vi "GUIQueueCluster.vi"() -> ()   [LabVIEW 2017]
uses:
  GUIQueueCluster.ctl
  GUIMessage.ctl
panel:
  in  "GUIQueueCluster":T1
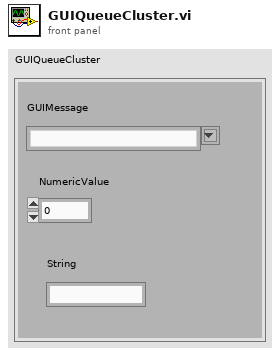
[diagram p1: front panel]
types:
  T1 = typedef "GUIQueueCluster.ctl" = cluster{"GUIMessage":T2, "NumericValue":dbl, "String":string}
  T2 = typedef "GUIMessage.ctl" = string
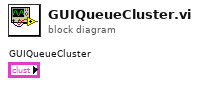
[diagram p0: block diagram]
diagram:
